vi "Get Stats.vi"(11 "Stats_DBL_CIF_U in":refnum<class "Stats_DBL_CIF_U.lvclass">) -> (0 "Min":dbl, 1 "Average":dbl, 2 "Max":dbl, 3 "Stats_DBL_CIF_U out":refnum<class "Stats_DBL_CIF_U.lvclass">, 5 "Iteration":u32)   [LabVIEW 2021, in "Stats_CIF_U.lvlib" / "Stats_DBL_CIF_U.lvclass"]
doc: "Get all the statistics for this data element. This data is also available via data accessors."
uses:
  Stats_DBL_CIF_U.lvclass
  Stats_DBL_CIF_U.lvclass/Stats_DBL_CIF_U.ctl
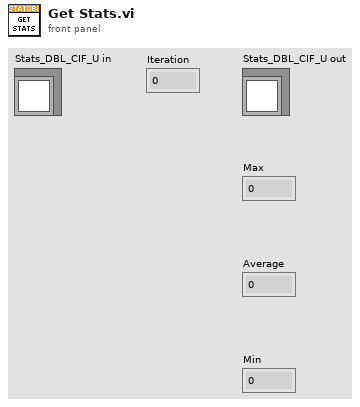
[diagram p1: front panel]
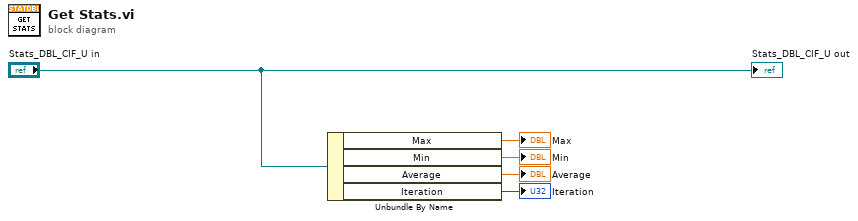
[diagram p0: block diagram]
diagram:
  n1 = Unbundle By Name("Stats_DBL_CIF_U in") -> ("Max"=→"Max":dbl, "Min"=→"Min":dbl, "Average"=→"Average":dbl, "Iteration"=→"Iteration":u32)
  "Stats_DBL_CIF_U out" <- "Stats_DBL_CIF_U in"
